vi "Teleop.vi"(10 "Match Info":T1={"Autonomous Elapsed Seconds"=0.0, "TeleOp Elapsed Seconds"=0.0, "Disabled Elapsed Seconds"=0.0, "Visited Autonomous"=FALSE, "Visited TeleOp"=FALSE, "Visited Disabled"=FALSE, "Autonomous Settings"={"Autonomous Style"=enum."Independent", "VI Refnum"=refnum}}, 11 "Call Context":T2) -> ()   [LabVIEW 2016]
doc: "This VI is called for each TeleOp packet received from the DS where the robot is not disabled. It is often used to read from the joysticks and update I/O or to update setpoints for timed control loops. It should complete and return within 20 milliseconds or it may miss DS packets."
uses:
  <vilib>/Rock Robotics/WPI/DriverStation/WPI_DriverStationDerivedRobotMode.ctl
  <vilib>/Rock Robotics/WPI/DriverStation/WPI_DriverStationMatch Info.ctl
  <vilib>/Rock Robotics/WPI/Utilities/WPI_GetSetVariantRefNum.vi
  <vilib>/Rock Robotics/WPI/Ultrasonic/WPI_SonarMB1010DigitalRefNum Registry Get.vi
  <vilib>/Rock Robotics/WPI/Ultrasonic/WPI_SonarMB1010DigitalGetRange.vi
  FRC SimulatedRSC/Positions.vi
panel:
  out "Encoder Position R":dbl
  out "Encoder Position L":dbl
  out "Gyro Angle":dbl format="%#_13g"
  in  "Set RPM":dbl=7000.0 format="%#_13g"
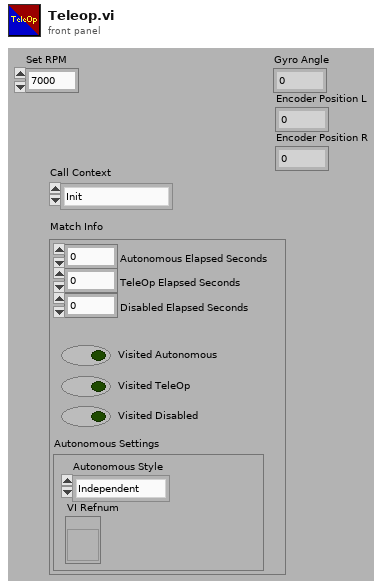
[diagram p1: front panel]
types:
  T1 = typedef "WPI_DriverStationMatch Info.ctl" = cluster{"Autonomous Elapsed Seconds":dbl, "TeleOp Elapsed Seconds":dbl, "Disabled Elapsed Seconds":dbl, "Visited Autonomous":bool, "Visited TeleOp":bool, "Visited Disabled":bool, "Autonomous Settings":cluster{"Autonomous Style":enum16{"Iterative", "Independent"}, "VI Refnum":refnum<vi>}}
  T2 = typedef "WPI_DriverStationDerivedRobotMode.ctl" = enum16{"Init", "Execute", "Stop"}
  T3 = typedef "WPI_JoystickDevRef.ctl" = cluster{"Device":T4}
  T4 = typedef "WPI_JoystickDeviceEnum.ctl" = enum16{"USB 0", "USB 1", "USB 2", "USB 3", "USB 4", "USB 5"}
  T5 = typedef "WPI_MotorControlDeviceRef.ctl" = cluster{"DeviceStatus":errorcluster, "Type":T6, "PWM":cluster{"PWM Channel":T7, "DeadBand":T8}, "CAN":cluster{"Device Number":u8, "SetOutput VI Ref":variant, "GetOutput VI Ref":variant, "Enable VI Ref":variant, "Disable VI Ref":variant, "Data":variant}, "Invert":bool}
  T6 = typedef "WPI_MotorControlType.ctl" = enum16{"PWM", "CAN"}
  T7 = typedef "FPGA_DIOPWMChannel.ctl" = enum8{"PWM 0", "PWM 1", "PWM 2", "PWM 3", "PWM 4", "PWM 5", "PWM 6", "PWM 7", "PWM 8", "PWM 9", "PWM MXP 0", "PWM MXP 1", "PWM MXP 2", "PWM MXP 3", "PWM MXP 4", "PWM MXP 5", "PWM MXP 6", "PWM MXP 7", "PWM MXP 8", "PWM MXP 9", "Invalid"}
  T8 = typedef "WPI_PWMDeadband.ctl" = cluster{"Name":string, "maxPositivePwm":i32, "minPositivePwm":i32, "centerPwm":i32, "maxNegativePwm":i32, "minNegativePwm":i32, "angularRange":u16}
  T9 = typedef "WPI_CANTalonSRX_GlobalStatus.ctl" = cluster{"Applied Throttle":dbl, "Module Enabled":bool, "CAN Error":errorcluster, "Closed Loop Error":dbl, "Forward Limit Switch Closed":bool, "Reverse Limit Switch Closed":bool, "Sensor Position":dbl, "Sensor Velocity":dbl, "Current":dbl, "Sticky Fault - Over Temp":bool, "Sticky Fault - Under Voltage":bool, "Sticky Fault - Forward Limit":bool, "Sticky Fault - Reverse Limit":bool, "Sticky Fault - Forward Soft Limit":bool, "Sticky Fault - Reverse Soft Limit":bool, "Brake is Enabled":bool, "Encoder Position":dbl, "Encoder Velocity":dbl, "Encoder Index Count":dbl, "Encoder A Pin State":bool, "Encoder B Pin State":bool, "Encoder Index Pin State":bool, "Analog In":dbl, "Analog In Velocity":dbl, "Temperature (C)":dbl, "Battery Voltage":dbl, "Control 5 Is Supported":bool, "Current Profile Slot Select":dbl, "Pos Div 8":bool, "Vel Div 4":bool, "Pulse Width Position":i32, "Pulse Width Velocity":i32, "Pulse Width Rise To Rise (us)":i32, "Pulse Width Rise To Fall (us)":i32, "Mot Prof Active Is Under Run":bool, "Mot Prof Active Has Under Run":bool, "Mot Prof Active Is Last":bool, "Mot Prof Active Velocity Only":bool, "Mot Prof Active Is Valid":bool, "Mot Prof Buffer Is Full":bool, "Mot Prof Active Profile Slot Select":i32, "Mot Prof NextID":i32, "Mot Prof Count":i32, "Mot Prof Active Velocity":dbl, "Mot Prof Active Position":dbl, "Mot Prof Output Enable":i32}
  T10 = typedef "WPI_SonarMB1010DigitalDeviceRef.ctl" = cluster{"CounterDevRef":T11, "Scaling factor (s/in)":dbl}
  T11 = typedef "WPI_CounterDevRef.ctl" = cluster{"DevStatus":errorcluster, "CntIndex":T12}
  T12 = typedef "FPGA_CounterCtrSystemIndex.ctl" = enum8{"Ctr 0", "Ctr 1", "Ctr 2", "Ctr 3", "Ctr 4", "Ctr 5", "Ctr 6", "Ctr 7", "Invalid"}
  T13 = typedef "WPI_GyroDevRef.ctl" = cluster{"DevStatus":errorcluster, "Analog Channel":T14, "Offset":dbl, "Gain (VoltsPerDegree/Second)":dbl, "Gyro Type":enum16{"Analog", "XRS450"}, "Handle":i32, "SPI Bus":T15, "Device Found":bool, "Sample Rate":dbl, "Calibrate On Open":bool}
  T14 = typedef "FPGA_AIChannel.ctl" = enum8{"AI 0", "AI 1", "AI 2", "AI 3", "AI MXP 0", "AI MXP 1", "AI MXP 2", "AI MXP 3", "Invalid"}
  T15 = typedef "spi_bus.ctl" = enum16{"SPI On-Board, CS0", "SPI On-Board, CS1", "SPI On-Board, CS2", "SPI On-Board, CS3", "SPI MXP", "Invalid"}
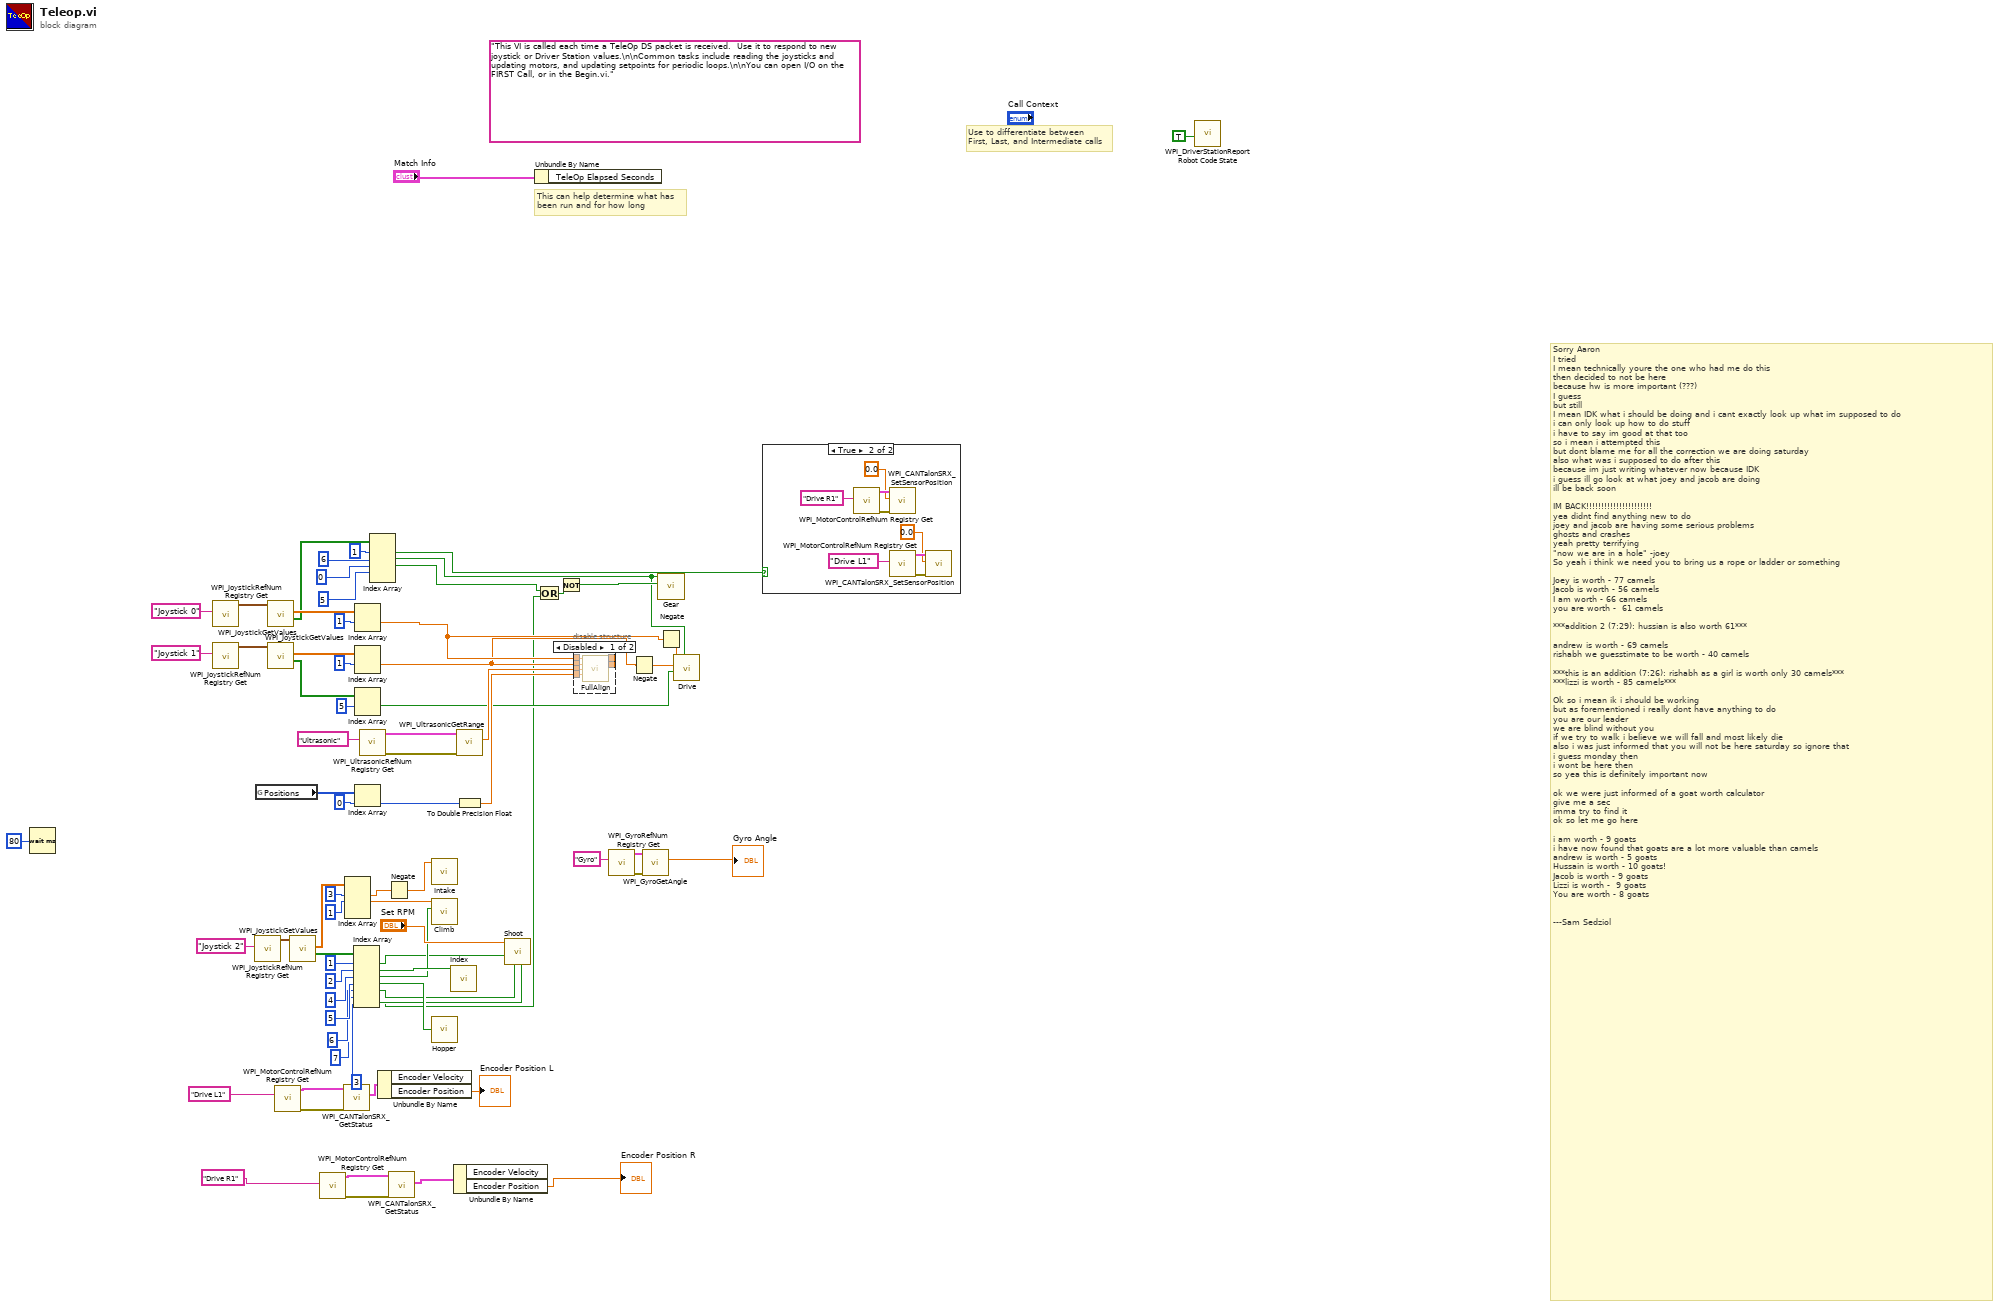
[diagram p0: block diagram]
diagram:
  (unwired) "This VI is called each time a TeleOp DS packet is received.  Use it to respond to new joystick or Driver Station values.\n\nCommon tasks include reading the joysticks and updating motors, and updating setpoints for periodic loops.\n\nYou can open I/O on the FIRST Call, or in the Begin.vi."
  # "Sorry Aaron\nI tried\nI mean technically youre the one who had me do this\nthen decided to not be here\nbecause hw is more important (???)\nI guess\nbut still\nI mean IDK what i should be doing and i cant exactly look up what im supposed to do\ni can only look up how to do stuff\ni have to say im good at that too\nso i mean i attempted this\nbut dont blame me for all the correction we are doing saturday\nalso what was i supposed to do after this\nbecause im just writing whatever now because IDK\ni guess ill go look at what joey and jacob are doing\nill be back soon\n\nIM BACK!!!!!!!!!!!!!!!!!!!!!!\nyea didnt find anything new to do\njoey and jacob are having some serious problems\nghosts and crashes\nyeah pretty terrifying\n\"now we are in a hole\" -joey\nSo yeah i think we need you to bring us a rope or ladder or something\n\nJoey is worth - 77 camels\nJacob is worth - 56 camels\nI am worth - 66 camels\nyou are worth -  61 camels \n\n***addition 2 (7:29): hussian is also worth 61***\n\nandrew is worth - 69 camels\nrishabh we guesstimate to be worth - 40 camels\n\n***this is an addition (7:26): rishabh as a girl is worth only 30 camels***\n***lizzi is worth - 85 camels***\n\nOk so i mean ik i should be working\nbut as forementioned i really dont have anything to do\nyou are our leader\nwe are blind without you\nif we try to walk i believe we will fall and most likely die\nalso i was just informed that you will not be here saturday so ignore that\ni guess monday then\ni wont be here then\nso yea this is definitely important now\n\nok we were just informed of a goat worth calculator\ngive me a sec \nimma try to find it\nok so let me go here\n\ni am worth - 9 goats\ni have now found that goats are a lot more valuable than camels\nandrew is worth - 5 goats\nHussain is worth - 10 goats! \nJacob is worth - 9 goats\nLizzi is worth -  9 goats\nYou are worth - 8 goats\n\n\n---Sam Sedziol"
  # "Use to differentiate between\nFirst, Last, and Intermediate calls"
  # "This can help determine what has\nbeen run and for how long"
  n1 = Wait (ms)(milliseconds to wait=u32 80) -> ()  [unwired: 1 out]
  n2 = call <vilib>:"WPI_JoystickRefNum Registry Get.vi"("refnum name"="Joystick 0") -> ("JoystickDevRef"=w48:T3)  [unwired: 1 in, 9 out]
  n3 = call <vilib>:"WPI_JoystickRefNum Registry Get.vi"("refnum name"="Joystick 1") -> ("JoystickDevRef"=w47:T3)  [unwired: 1 in, 9 out]
  n4 = call <vilib>:"WPI_JoystickRefNum Registry Get.vi"("refnum name"="Joystick 2") -> ("JoystickDevRef"=w68:T3)  [unwired: 1 in, 9 out]
  n5 = global read "Positions.vi" "Positions"() -> (w49:i32[])
  n6 = call <vilib>:"WPI_JoystickGetValues.vi"("JoystickDevRef"=w48) -> ("Buttons"=w64:bool[], "Axes"=w71:dbl[])  [unwired: 6 in, 3 out]
  n7 = call <vilib>:"WPI_JoystickGetValues.vi"("JoystickDevRef"=w47) -> ("Buttons"=w65:bool[], "Axes"=w70:dbl[])  [unwired: 6 in, 3 out]
  n8 = call <vilib>:"WPI_MotorControlRefNum Registry Get.vi"("refnum name"="Drive L1") -> ("error out"=w5:errorcluster, "MotorControlDevRef"=w10:T5)  [unwired: 9 in]
  n9 = call <vilib>:"WPI_JoystickGetValues.vi"("JoystickDevRef"=w68) -> ("Buttons"=w66:bool[], "Axes"=w67:dbl[])  [unwired: 6 in, 3 out]
  n10 = call <vilib>:"WPI_MotorControlRefNum Registry Get.vi"("refnum name"="Drive R1") -> ("error out"=w8:errorcluster, "MotorControlDevRef"=w9:T5)  [unwired: 9 in]
  n11 = call <vilib>:"WPI_CANTalonSRX_GetStatus.vi"("error in (no error)"=w5, "CAN Talon SRX Ref"=w10) -> ("Talon SRX Status"=w7:T9)  [unwired: 7 in, 2 out]
  n12 = Index Array(array=w67, index #1=3 ("index"), index #2=1 ("index")) -> (element #1=w61:dbl, element #2=w51:dbl)  [unwired: 2 in, 2 out]
  n13 = Index Array(array=w66, index #1=1 ("index"), index #2=2 ("index"), index #3=4 ("index"), index #4=5 ("index"), index #5=6 ("index"), index #6=7 ("index"), index #7=3 ("index")) -> (element #1=w25:bool, element #2=w50:bool, element #3=w33:bool, element #4=w32:bool, element #5=w22:bool, element #6=w21:bool, element #7=w16:bool)
  n14 = Index Array(array=w71, index #1=1 ("index")) -> (element #1=w27:dbl)  [unwired: 1 in, 1 out]
  n15 = Index Array(array=w70, index #1=1 ("index")) -> (element #1=w26:dbl)  [unwired: 1 in, 1 out]
  n16 = Index Array(array=w65, index #1=5 ("index")) -> (element #1=w28:bool)  [unwired: 1 in, 1 out]
  n17 = Index Array(array=w49, index=0) -> (element=w53:i32)
  n18 = call-poly <vilib>:"WPI_UltrasonicRefNum Registry Get.vi"("refnum name"="Ultrasonic") -> ("error out"=w59:errorcluster, "SonarMB1010DigitalDevRef"=w60:T10)  [unwired: 9 in]
  n19 = Index Array(array=w64, index #1=1 ("index"), index #2=6 ("index"), index #3=0 ("index"), index #4=5 ("index")) -> (element #1=w56:bool, element #2=w11:bool, element #3=w20:bool)  [unwired: 1 in, 2 out]
  n20 = Unbundle By Name(w7) -> ("Encoder Position"=→"Encoder Position L":dbl)  [unwired: 1 out]
  n21 = Negate(x=w61) -> (-x=w42:dbl)
  n22 = call <vilib>:"WPI_CANTalonSRX_GetStatus.vi"("error in (no error)"=w8, "CAN Talon SRX Ref"=w9) -> ("Talon SRX Status"=w6:T9)  [unwired: 7 in, 2 out]
  n23 = call "Intake.vi"("Effort"=w42) -> ()  [unwired: 11 in]
  n24 = call "Climb.vi"("Backwards?"=w33, "Effort"=w51) -> ()  [unwired: 10 in]
  n25 = call "Hopper.vi"("Hopper?"=w32) -> ()  [unwired: 4 in]
  n26 = call "Index.vi"("Index?"=w50) -> ()  [unwired: 11 in]
  n27 = Unbundle By Name(w6) -> ("Encoder Position"=→"Encoder Position R":dbl)  [unwired: 1 out]
  n28 = call-poly <vilib>:"WPI_UltrasonicGetRange.vi"("error in"=w59, "SonarMB1010DigitalDevRef"=w60) -> ("Distance"=w57:dbl)  [unwired: 7 in, 2 out]
  n29 = To Double Precision Float(number=w53) -> (double precision float=w52:dbl)
  n30 = call "Shoot.vi"("Icrement Up"=w21, "Icrement Down"=w22, "Override?"=w25, "Set RPM"="Set RPM") -> ()  [unwired: 8 in]
  n31 = Unbundle By Name("Match Info") -> ()  [unwired: 1 out]
  n32 = Or(x=w20, y=w16) -> (x .or. y?=w19:bool)
  n33 = Not(x=w19) -> (.not. x?=w18:bool)
  n34 = disable-structure shown="Disabled" {
    disable-tunnel: w27 -> [w80 _]
    disable-tunnel: w26 -> [w79 _]
    disable-tunnel: w57 -> [w78 _]
    disable-tunnel: w52 -> [w77 _]
    disable-tunnel: [w76 _] -> _
    disable-tunnel: [w75 _] -> _
    frame Disabled {
      n35 = call "FullAlign.vi"("Joystick 0"=w80, "Joystick 1"=w79, "Distance"=w78, "Angle"=w77) -> ("Right Motor"=w75:dbl, "Left Motor"=w76:dbl)  [unwired: 9 in, 1 out]
    }
    frame Enabled {
    }
  }
  n36 = call <vilib>:"WPI_GyroRefNum Registry Get.vi"("refnum name"="Gyro") -> ("error out"=w15:errorcluster, "GyroDevRef"=w14:T13)  [unwired: 9 in]
  n37 = Negate(x=w26) -> (-x=w38:dbl)
  n38 = call <vilib>:"WPI_GyroGetAngle.vi"("error in"=w15, "GyroDevRef"=w14) -> ("Angle"=→"Gyro Angle":dbl)  [unwired: 5 in, 4 out]
  n39 = call "Gear.vi"("Gear1?"=w18, "Gear0?"=w11) -> ()  [unwired: 10 in]
  n40 = Negate(x=w27) -> (-x=w39:dbl)
  n41 = call "Drive.vi"("Slow?"=w11, "SwitchDir"=w28, "Drive L"=w38, "Drive R"=w39) -> ()  [unwired: 8 in]
  n42 = case shown="True" w56 {
    frame False {
    }
    frame True {
      n43 = call <vilib>:"WPI_MotorControlRefNum Registry Get.vi"("refnum name"="Drive R1") -> ("error out"=w83:errorcluster, "MotorControlDevRef"=w82:T5)  [unwired: 9 in]
      n44 = call <vilib>:"WPI_CANTalonSRX_SetSensorPosition.vi"("error in (no error)"=w83, "New Sensor Position"=0.0, "CAN Talon SRX Ref"=w82) -> ()  [unwired: 7 in, 2 out]
      n45 = call <vilib>:"WPI_MotorControlRefNum Registry Get.vi"("refnum name"="Drive L1") -> ("error out"=w85:errorcluster, "MotorControlDevRef"=w86:T5)  [unwired: 9 in]
      n46 = call <vilib>:"WPI_CANTalonSRX_SetSensorPosition.vi"("error in (no error)"=w85, "New Sensor Position"=0.0, "CAN Talon SRX Ref"=w86) -> ()  [unwired: 7 in, 2 out]
    }
  }
  n47 = call <vilib>:"WPI_DriverStationReport Robot Code State.vi"("TeleOp"=TRUE ("Autonomous")) -> ()  [unwired: 10 in, 1 out]
